vi "Build State String with Arguments Plus.vi"(3 "Source (\"\")":string, 4 "Arguments (\"\")":string, 5 "State":string) -> (1 "State with Arguments":string)   [LabVIEW 2020]
doc: "Builds a state string that contains arguments for the JKI State Machine.\n<B>For Example:</B> If State = A and Arguments = B then State with Arguments = A >> B\n\nFor instructions on how to use the JKI State Machine, examples and video tutorials, visit:\nhttp://jkisoft.com/state-machine/\n\n<B>Inputs:</B>\n <B>State:</B> The State string that requires the argument.\n <B>Arguments:</B> The Argument string to add to the state. The default is an empty string. If Argument is an empty string then State will be returned to the output. <B>Note:</B> The arguments input must not contain any unprintable characters like linefeed or carriage return.\n\n<B>Outputs:</B>\n <B>State with Arguments:</B> This output returns the new string that contains the State and the Argument. <B>For Example:</B> If State = A and Arguments = B then State with Arguments = A >> B\n\nJKI State Machine™ 2018.0.7.45\nhttp://jki.net/state-machine/\nCopyright (C) 2005-2018, JKI <info@jki.net>\nALL RIGHTS RESERVED"
panel:
  # "For instructions on how to use the JKI State Machine, examples and video tutorials, visit:\nhttp://jki.net/state-machine/\n\nJKI State Machine™\nhttp://jki.net/state-machine/\nCopyright (C) 2005-2017, JKI <info@jki.net>\nALL RIGHTS RESERVED"
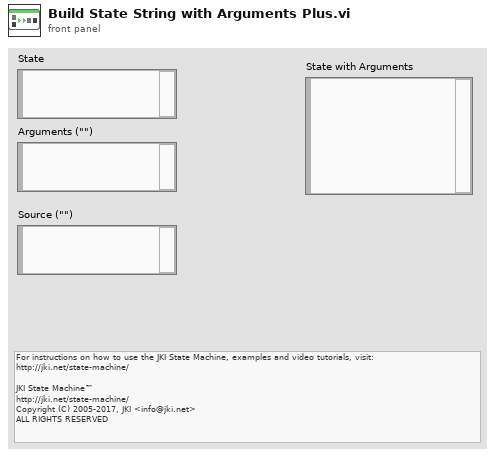
[diagram p1: front panel]
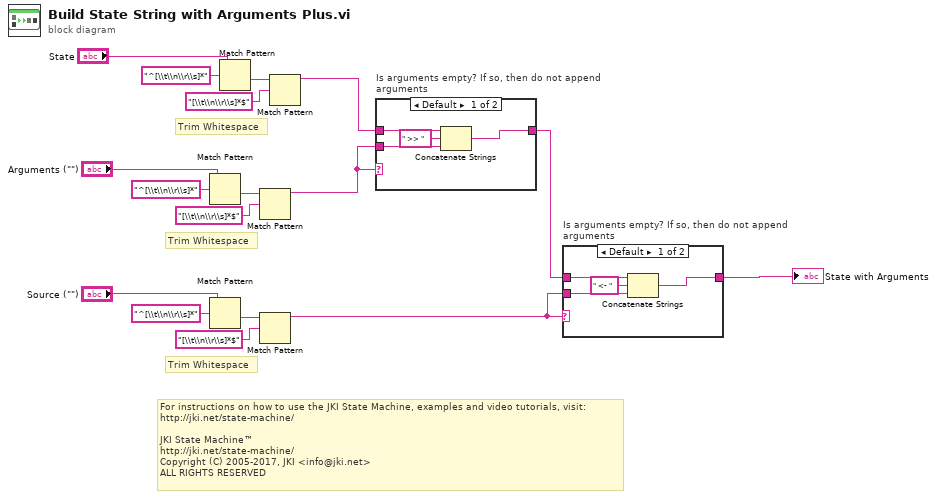
[diagram p0: block diagram]
diagram:
  # "Trim Whitespace"
  # "For instructions on how to use the JKI State Machine, examples and video tutorials, visit:\nhttp://jki.net/state-machine/\n\nJKI State Machine™\nhttp://jki.net/state-machine/\nCopyright (C) 2005-2017, JKI <info@jki.net>\nALL RIGHTS RESERVED"
  # "Trim Whitespace"
  # "Trim Whitespace"
  n1 = Match Pattern(string="Arguments (\"\")", regular expression="^[\\t\\n\\r\\s]*") -> (after substring=w11:string)  [unwired: 1 in, 3 out]
  n2 = Match Pattern(string="Source (\"\")", regular expression="^[\\t\\n\\r\\s]*") -> (after substring=w6:string)  [unwired: 1 in, 3 out]
  n3 = Match Pattern(string="State", regular expression="^[\\t\\n\\r\\s]*") -> (after substring=w16:string)  [unwired: 1 in, 3 out]
  n4 = Match Pattern(string=w11, regular expression="[\\t\\n\\r\\s]*$") -> (before substring=w8:string)  [unwired: 1 in, 3 out]
  n5 = Match Pattern(string=w6, regular expression="[\\t\\n\\r\\s]*$") -> (before substring=w2:string)  [unwired: 1 in, 3 out]
  n6 = Match Pattern(string=w16, regular expression="[\\t\\n\\r\\s]*$") -> (before substring=w13:string)  [unwired: 1 in, 3 out]
  n7 = case "Is arguments empty? If so, then do not append arguments" shown="Default" w8 {
    tunnel: [w18 w22] -> w3
    tunnel: w13 -> [w21 w22]
    tunnel: w8 -> [w19 _]
    frame Default {
      n8 = Concatenate Strings(w21, " >> " ("string"), w19) -> (w18:string)
    }
    frame "" {
    }
  }
  n9 = case "Is arguments empty? If so, then do not append arguments" shown="Default" w2 {
    tunnel: [w23 w27] -> w1
    tunnel: w3 -> [w26 w27]
    tunnel: w2 -> [w24 _]
    frame Default {
      n10 = Concatenate Strings(w26, " <- " ("string"), w24) -> (w23:string)
    }
    frame "" {
    }
  }
  "State with Arguments" <- w1
